vi "ICP waveform generator.vi"() -> ()   [LabVIEW 2015]
uses:
  <vilib>/express/express shared/transition.llb/Dynamic To Waveform Array.vi
  <vilib>/express/express signal manip/GetorSetDDTAttributes/Set DDT Attributes/SetT0.vi
  <vilib>/express/express shared/transition.llb/Waveform Array To Dynamic.vi
  <vilib>/express/express signal manip/GetorSetDDTAttributes/Set DDT Attributes/Set DDT Properties.xnode
panel:
  out "y value":dbl
  out "x value":dbl
  in  "stop":bool
  out "test ICP input":cluster{i32[], dbl[]}(graph)
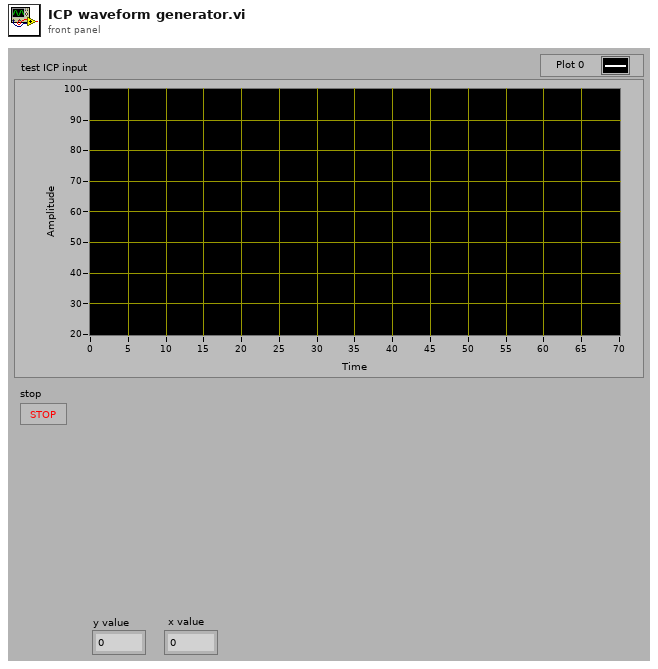
[diagram p1: front panel]
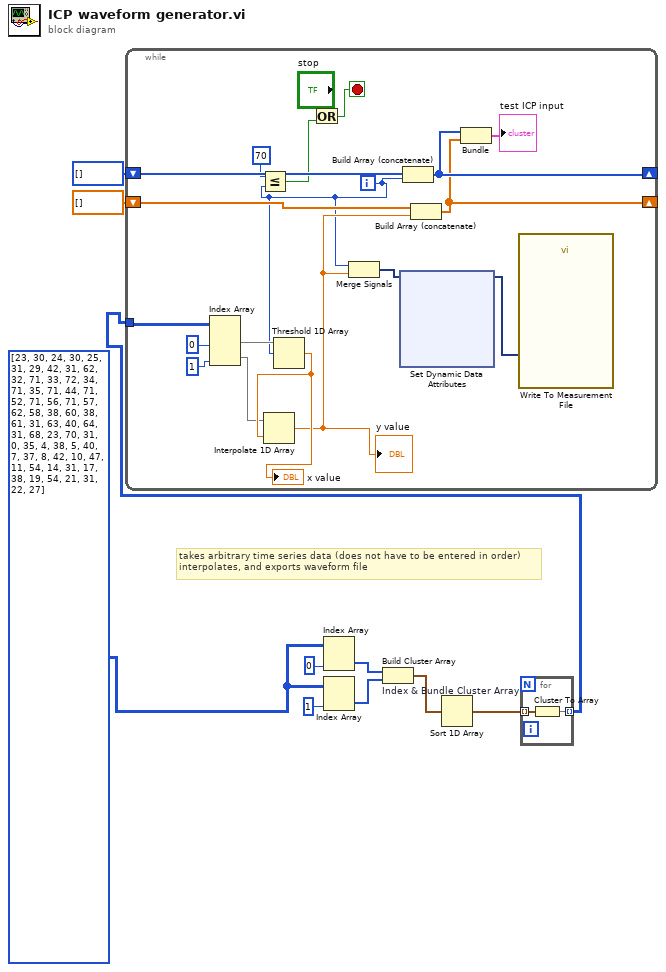
[diagram p0: block diagram]
diagram:
  w2 = i32[][] [[23, 30], [24, 30], [25, 31], [29, 42], [31, 62], [32, 71], [33, 72], [34, 71], [35, 71], [44, 71], [52, 71], [56, 71], [57, 62], [58, 38], [60, 38], [61, 31], [63, 40], [64, 31], [68, 23], [70, 31], [0, 35], [4, 38], [5, 40], [7, 37], [8, 42], [10, 47], [11, 54], [14, 31], [17, 38], [19, 54], [21, 31], [22, 27]]
  # "takes arbitrary time series data (does not have to be entered in order)\ninterpolates, and exports waveform file"
  n1 = Index Array(array=w2, index (col)=0) -> (element=w8:i32[])  [unwired: 1 in]
  n2 = Index Array(array=w2, index (col)=1) -> (element=w7:i32[])  [unwired: 1 in]
  n3 = Build Cluster Array "Index & Bundle Cluster Array"(w8, w7) -> (w6:cluster{i32, i32}[])
  n4 = Sort 1D Array(array=w6) -> (sorted array=w5:cluster{i32, i32}[])
  n5 = for {
    tunnel: w5 -> [w12] mode=indexing
    tunnel: [w11] -> w1 mode=indexing
    n6 = Cluster To Array(cluster=w12) -> (array=w11:i32[])
  }
  n7 = while {
    shift-right: [w29] -> _
    shift-left: dbl[] [] -> [w16]
    shift-right: [w30] -> _
    shift-left: i32[] [] -> [w31]
    tunnel: w1 -> [w18]
    i -> [w13]
    stop <- w22 stop-if-true
    n8 = Index Array(array=w18, index (col) #1=0 ("index (col)"), index (col) #2=1 ("index (col)")) -> (element #1=w20:i32[], element #2=w19:i32[])  [unwired: 2 in]
    n9 = Less Or Equal?(x=70 ("index (col)"), y=w13) -> (x <= y?=w23:bool)
    n10 = Threshold 1D Array(2:w13, 3:w20) -> (0:w25:dbl)  [unwired: 1 in]
    "x value" <- w25
    n11 = Interpolate 1D Array(1:w25, 2:w19) -> (0:w14:dbl)
    "y value" <- w14
    n12 = Or(x="stop", y=w23) -> (x .or. y?=w22:bool)
    n13 = Merge Signals(w13, w14) -> (w15:dynamicdata)
    n14 = xnode "Set Dynamic Data Attributes"("Signals In"=w15) -> ("Signals Out"=w17:dynamicdata)  [unwired: 3 in, 1 out]
    n15 = Build Array (concatenate)(w31, w13) -> (w30:i32[])
    n16 = Build Array (concatenate)(w16, w14) -> (w29:dbl[])
    n17 = Bundle(w30, w29) -> (→"test ICP input":cluster{i32[], dbl[]})  [unwired: 1 in]
    n18 = call "Write To Measurement File"("Signals"=w17) -> ()  [unwired: 16 in, 3 out]
  }
